vi "Get Count.vi"(8 "error in":errorcluster, 11 "Sub Objects Dictionary in":refnum<class "Sub Objects Dictionary.lvclass">) -> (0 "error out":errorcluster, 2 "Count":i32, 3 "Sub Objects Dictionary out":refnum<class "Sub Objects Dictionary.lvclass">)   [LabVIEW 2020, in "CANopen.lvlib" / "Sub Objects Dictionary.lvclass"]
doc: "Gets the number of Sub Objects contained in the Dictionary."
uses:
  Sub Objects Dictionary.lvclass
  Sub Objects Dictionary.lvclass/Sub Objects Dictionary.ctl
  Ordered-Dictionary/Ordered Object Dictionary/Source/Ordered Object Dictionary.lvclass
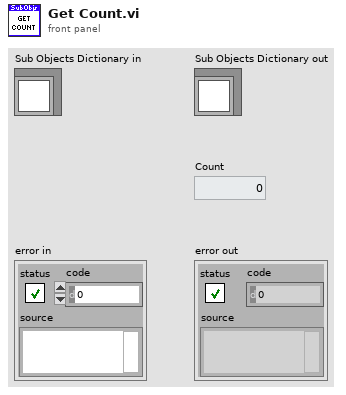
[diagram p1: front panel]
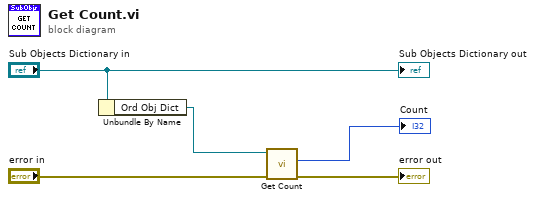
[diagram p0: block diagram]
diagram:
  n1 = Unbundle By Name("Sub Objects Dictionary in") -> ("Ord Obj Dict"=w3:refnum<class "Ordered Object Dictionary.lvclass">)
  n2 = call "Get Count.vi"("error in"="error in", "Ordered Object Dictionary in"=w3) -> ("error out"=→"error out":errorcluster, "Count"=→"Count":i32)  [unwired: 7 in, 1 out]
  "Sub Objects Dictionary out" <- "Sub Objects Dictionary in"
